vi "Function.vi"(8 "error in (no error)":errorcluster, 10 "Value":u16, 11 "Two Terminal in":refnum<class "Decrement_U16.lvclass">) -> (0 "error out":errorcluster, 2 "Result":u16, 3 "Two Terminal out":refnum<class "Decrement_U16.lvclass">)   [LabVIEW 2021, in "Decrement_U16.lvclass"]
uses:
  Decrement_U16.lvclass
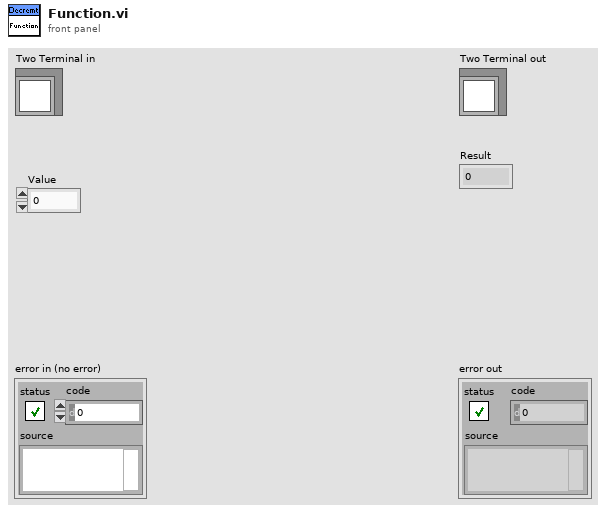
[diagram p1: front panel]
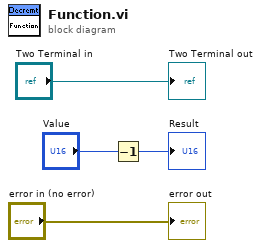
[diagram p0: block diagram]
diagram:
  n1 = Decrement(x="Value") -> (x-1=→"Result":u16)
  "error out" <- "error in (no error)"
  "Two Terminal out" <- "Two Terminal in"
